vi "tm_getdcimgframe_40.vi"(6 "View":i32(ring) items=["default"=0, "view 1"=1048576, "view 2"=2097152, "view 3"=3145728, "view 4"=4194304], 7 "Options":i32(ring) items=["no option"=0, "high contrast"=16], 8 "error in (no error)":errorcluster, 10 "Frame Index":i32=-1, 11 "File Handle in":u32) -> (0 "error out":errorcluster, 1 "Timestamp":dbl, 2 "Data":u16[][](array[numeric]), 3 "File Handle out":u32)   [LabVIEW 2023]
uses:
  tmcamcon.dll
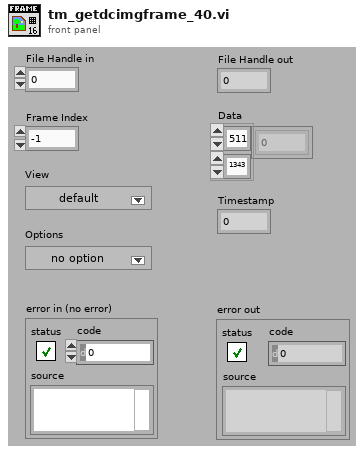
[diagram p1: front panel]
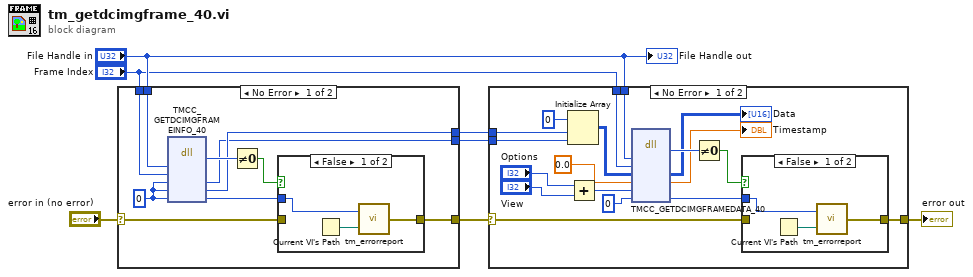
[diagram p0: block diagram]
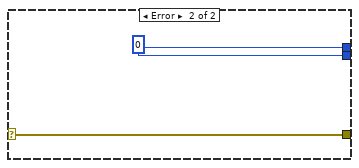
[diagram p5: hidden frame]
diagram:
  n1 = case shown="No Error" "error in (no error)" {
    selector: "error in (no error)" -> [w11 w23]
    tunnel: [w8 w23] -> w6
    tunnel: "File Handle in" -> [w16 _]
    tunnel: [w12 w22] -> w3
    tunnel: [w13 w22] -> w4
    tunnel: "Frame Index" -> [w14 _]
    frame No Error {
      w15 = 0 ("Erval")
      n2 = dll-call lib="tmcamcon.dll" fn="TMCC_GETDCIMGFRAMEINFO_40"("index"=w16, "frameindex"=w14, "width"=w15, "height"=w15, "Erval"=w15) -> ("return type"=w17:u32, "width"=w12:i32, "height"=w13:i32, "Erval"=w10:i32)  [unwired: 5 in, 2 out]
      n3 = Not Equal To 0?(x=w17) -> (x != 0?=w9:bool)
      n4 = case shown="False" w9 {
        tunnel: w11 -> [_ w21]
        tunnel: [w19 w21] -> w8
        tunnel: w10 -> [w18 _]
        frame False {
          n5 = Current VI's Path() -> (path=w20:path)
          n6 = call "tm_errorreport.vi"("Source"=w20, "Error"=w18) -> ("error out"=w19:errorcluster)
        }
        frame True {
        }
      }
    }
    frame Error {
      w22 = 0 ("buf")
    }
  }
  n7 = case shown="No Error" w6 {
    selector: w6 -> [w30 w46]
    tunnel: [w27 w46] -> w2
    tunnel: "File Handle in" -> [w40 _]
    tunnel: w4 -> [w38 _]
    tunnel: w3 -> [w37 _]
    tunnel: "Frame Index" -> [w34 _]
    frame No Error {
      n8 = Initialize Array(u16 0 ("buf"), w38, w37) -> (w36:u16[][])
      n9 = Add(x="Options", y="View") -> (x+y=w26:i32)
      n10 = dll-call lib="tmcamcon.dll" fn="TMCC_GETDCIMGFRAMEDATA_40"("index"=w40, "frame"=w34, "imgarray"=w36, "timestamp"=0.0 ("Erval"), "option"=w26, "Erval"=0) -> ("return type"=w41:u32, "imgarray"=→"Data":u16[][], "timestamp"=→"Timestamp":dbl, "Erval"=w29:i32)  [unwired: 6 in, 2 out]
      n11 = Not Equal To 0?(x=w41) -> (x != 0?=w28:bool)
      n12 = case shown="False" w28 {
        tunnel: w30 -> [_ w45]
        tunnel: [w43 w45] -> w27
        tunnel: w29 -> [w42 _]
        frame False {
          n13 = Current VI's Path() -> (path=w44:path)
          n14 = call "tm_errorreport.vi"("Source"=w44, "Error"=w42) -> ("error out"=w43:errorcluster)
        }
        frame True {
        }
      }
    }
    frame Error {
    }
  }
  "error out" <- w2
  "File Handle out" <- "File Handle in"
